vi "NodeFileNameGen.vi"(9 "Node Info in":T2 {"Year" format="%02d"; "Patient Number" format="%03d"; "Node Number" format="%02d"}, 11 "Location":T1) -> (0 "Other Box Visible?":bool, 1 "Node Info out":T2 {"Year" format="%02d"; "Patient Number" format="%03d"; "Node Number" format="%02d"}, 2 "SavePathOut":path, 4 "PatientFileName":string)   [LabVIEW 2022 SP3]
uses:
  LymphNodeInfo.ctl
  TissueTypeScan.ctl
  ScanningControl/-ScanSystem/Controls/location.ctl
  ScanningControl/Motion Controllers/-MotionRoutines/MotionGlobals.vi
  PatientGlobals.vi
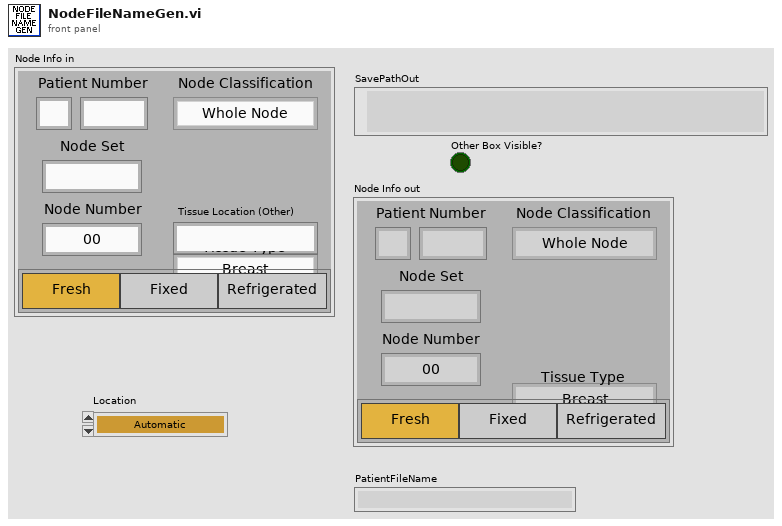
[diagram p1: front panel]
types:
  T1 = typedef "location.ctl" = enum16{"Automatic", "WCM Main", "Hawaii", "Columbia MM3000", "Columbia  NI System", "NYU", "RRI 2", "UHI Allen", "CUMC RT", "Chiba", "Stony Brook", "WCM Microscopy", "WCM Aeoretch", "WCM Optics Lab", "WCM Main 2Axis", "WCM Rotation", "WCM SAM SMAC", "SERI GP"}
  T2 = typedef "LymphNodeInfo.ctl" = cluster{"Patient Number":u32, "Node Set":string, "Node Number":u32, "Tissue Type":T3, "Tissue Location (Other)":string, "Node Classification":enum16{"Whole Node", "Piece A", "Piece B", "Piece C"}, "Fresh?":enum32{"Fresh?", "Fixed?", "Refrigerated?"}, "Year":u32}
  T3 = typedef "TissueTypeScan.ctl" = enum16{"Breast", "Gastric", "Stomach", "Rectal", "Colon", "Head & Neck", "Other"}
  T4 = enum16{"Whole Node", "Piece A", "Piece B", "Piece C"}
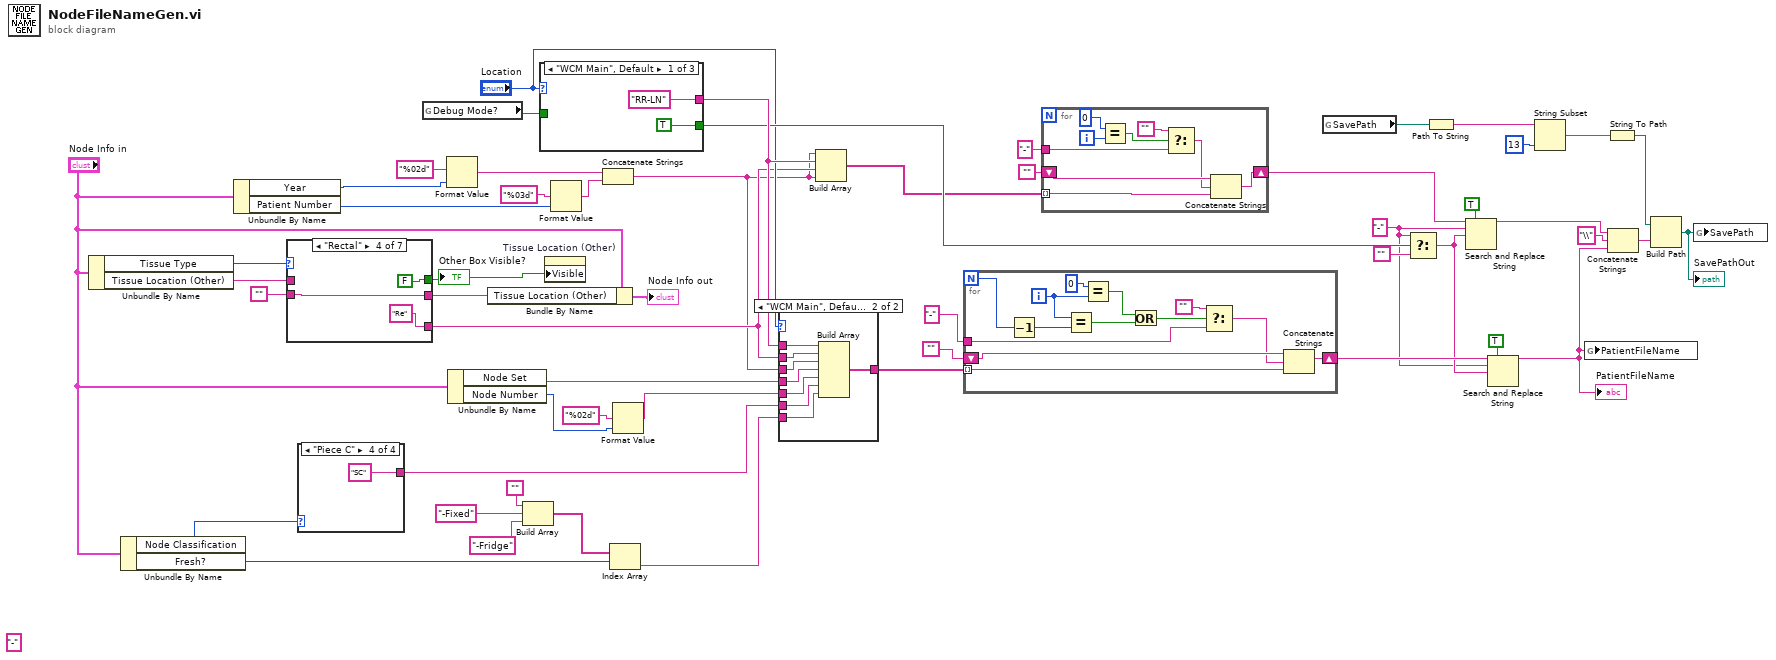
[diagram p0: block diagram]
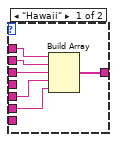
[diagram p2: hidden frame]
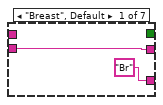
[diagram p3: hidden frame]
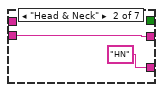
[diagram p4: hidden frame]
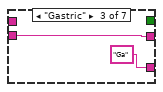
[diagram p5: hidden frame]
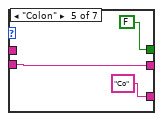
[diagram p6: hidden frame]
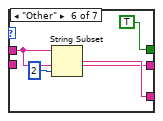
[diagram p7: hidden frame]
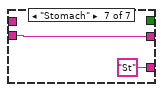
[diagram p8: hidden frame]
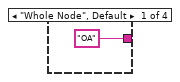
[diagram p9: hidden frame]
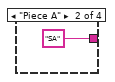
[diagram p10: hidden frame]
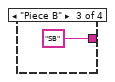
[diagram p11: hidden frame]
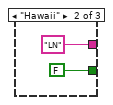
[diagram p12: hidden frame]
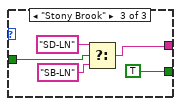
[diagram p13: hidden frame]
diagram:
  w15 = "-"
  (unwired) "-" ("string")
  n1 = Unbundle By Name("Node Info in") -> ("Tissue Type"=w51:T3, "Tissue Location (Other)"=w52:string)
  n2 = Unbundle By Name("Node Info in") -> ("Node Classification"=w7:T4, "Fresh?"=w8:enum32{"Fresh?", "Fixed?", "Refrigerated?"})
  n3 = Unbundle By Name("Node Info in") -> ("Year"=w6:u32, "Patient Number"=w5:u32)
  n4 = case shown="\"Rectal\"" w51 {
    tunnel: ["Br" "HN" "Ga" "Re" "Co" w70 "St" ("Tissue Location (Other)")] -> w12
    tunnel: w52 -> [_ _ _ _ _ w68 _]
    tunnel: [w55 w57 w59 w62 w65 w68 w72] -> w53
    tunnel: "" ("Value") -> [w55 w57 w59 w62 w65 _ w72]
    tunnel: [_ _ _ FALSE ("Visible") FALSE ("Visible") TRUE ("Visible") _] -> w36
    frame "Breast", Default {
    }
    frame "Head & Neck" {
    }
    frame "Gastric" {
    }
    frame "Rectal" {
    }
    frame "Colon" {
    }
    frame "Other" {
      n5 = String Subset(string=w68, length (rest)=2 ("length (rest)")) -> (substring=w70:string)  [unwired: 1 in]
    }
    frame "Stomach" {
    }
  }
  "Other Box Visible?" <- w36
  n6 = case shown="\"Piece C\"" w7 {
    tunnel: ["OA" "SA" "SB" "SC"] -> w47
    frame "Whole Node", Default {
    }
    frame "Piece A" {
    }
    frame "Piece B" {
    }
    frame "Piece C" {
    }
  }
  n7 = global read "MotionGlobals.vi" "Debug Mode?"() -> (w13:bool)
  n8 = Format Value(format string="%02d", value (0)=w6) -> (output string=w10:string)  [unwired: 1 in]
  n9 = Unbundle By Name("Node Info in") -> ("Node Set"=w4:string, "Node Number"=w1:u32)
  n10 = Bundle By Name(cluster="Node Info in", "Tissue Location (Other)"=w53) -> (→"Node Info out":T2)
  n11 = Build Array("" ("t"), "-Fixed" ("string"), "-Fridge" ("string")) -> (w32:string[])
  n12 = case shown="\"WCM Main\", Default" "Location" {
    tunnel: ["RR-LN" "LN" w81] -> w48
    tunnel: [TRUE FALSE TRUE] -> w28
    tunnel: w13 -> [_ _ w83]
    frame "WCM Main", Default {
    }
    frame "Hawaii" {
    }
    frame "Stony Brook" {
      n13 = Select(t="SD-LN", s=w83, f="SB-LN") -> (s? t:f=w81:string)
    }
  }
  n14 = property on="Tissue Location (Other)" class="Str"("Visible"=w36) -> ()  [unwired: 2 in, 2 out]
  n15 = Format Value(format string="%03d", value (0)=w5) -> (output string=w9:string)  [unwired: 1 in]
  n16 = Concatenate Strings(w10, w9) -> (w2:string)
  n17 = Index Array(array=w32, index=w8) -> (element=w31:string)
  n18 = Format Value(format string="%02d", value (0)=w1) -> (output string=w49:string)  [unwired: 1 in]
  n19 = case shown="\"WCM Main\", Default" "Location" {
    tunnel: w12 -> [w90 w99]
    tunnel: w4 -> [_ w98]
    tunnel: w49 -> [w86 w97]
    tunnel: w48 -> [w91 w96]
    tunnel: w47 -> [w88 w95]
    tunnel: w31 -> [_ w94]
    tunnel: [w87 w93] -> w30
    tunnel: w2 -> [w89 w92]
    frame "Hawaii" {
      n20 = Build Array(w91, w90, w89, w86, w88) -> (w87:string[])
    }
    frame "WCM Main", Default {
      n21 = Build Array(w96, w99, w92, w98, w97, w95, w94) -> (w93:string[])
    }
  }
  n22 = Build Array(w2, w48, w12, w2) -> (w23:string[])
  n23 = for {
    N -> [w103]
    tunnel: w30 -> [w110] mode=indexing
    tunnel: "-" -> [w106]
    shift-right: [w112] -> w26
    shift-left: "" -> [w111]
    i -> [w102]
    n24 = Decrement(x=w103) -> (x-1=w101:i32)
    n25 = Equal?(x=w102, y=w101) -> (x = y?=w100:bool)
    n26 = Equal?(x=0, y=w102) -> (x = y?=w107:bool)
    n27 = Or(x=w107, y=w100) -> (x .or. y?=w104:bool)
    n28 = Select(t="", s=w104, f=w106) -> (s? t:f=w108:string)
    n29 = Concatenate Strings(w111, w108, w110) -> (w112:string)
  }
  n30 = for {
    tunnel: w23 -> [w119] mode=indexing
    tunnel: "-" -> [w116]
    shift-right: [w121] -> w20
    shift-left: "" -> [w120]
    i -> [w113]
    n31 = Equal?(x=0, y=w113) -> (x = y?=w114:bool)
    n32 = Select(t="", s=w114, f=w116) -> (s? t:f=w117:string)
    n33 = Concatenate Strings(w120, w117, w119) -> (w121:string)
  }
  n34 = global read "MotionGlobals.vi" "SavePath"() -> (w38:path)
  n35 = Select(t=w15, s=w28, f="") -> (s? t:f=w18:string)
  n36 = Path To String(path=w38) -> (string=w42:string)
  n37 = Search and Replace String(replace all?=TRUE ("replace all? (F)"), input string=w20, search string=w15, replace string=w18) -> (result string=w21:string)  [unwired: 4 in, 3 out]
  n38 = Search and Replace String(replace all?=TRUE ("replace all? (F)"), input string=w26, search string=w15, replace string=w18) -> (result string=w25:string)  [unwired: 4 in, 3 out]
  "PatientFileName" <- w25
  n39 = String Subset(string=w42, length (rest)=13 ("length (rest)")) -> (substring=w40:string)  [unwired: 1 in]
  n40 = global write "PatientGlobals.vi" "PatientFileName"(w25) -> ()
  n41 = String To Path(string=w40) -> (path=w39:path)
  n42 = Concatenate Strings(w21, "\\" ("string"), w25) -> (w43:string)
  n43 = Build Path(base path=w39, name or relative path=w43) -> (appended path=w37:path)
  "SavePathOut" <- w37
  n44 = global write "MotionGlobals.vi" "SavePath"(w37) -> ()
